vi "Create Key Index Map.vi"(6 "Key Map Transposed Primitive":refnum<class "2D Array u32.lvclass">, 8 "error in (no error)":errorcluster, 9 "Key Map Primitive":refnum<class "2D Array u32.lvclass">, 10 "Reduced Keys for Each line Profile":refnum<class "1D Array u32.lvclass">, 11 "Unique Keys":refnum<class "1D Array u32.lvclass">) -> (0 "error out":errorcluster, 3 "Key Line Profile Indexes":refnum<class "1D Array u32.lvclass">)   [LabVIEW 2024, in "G2CPU Line Profile.lvlib"]
uses:
  G2CPU Line Profile.lvlib
  <vilib>/Natan Biesmans/G2CPU GPU and CPU HPC Toolkit/G2CPU Libraries/Arrays/2DArray/u32/2D Array u32.lvclass
  C:/Program Files/National Instruments/LabVIEW 2025/vi.lib/Natan Biesmans/G2CPU GPU and CPU HPC Toolkit/G2CPU Libraries/Arrays/Array/Array Prototype.lvclass
  <vilib>/Natan Biesmans/G2CPU GPU and CPU HPC Toolkit/G2CPU Libraries/Arrays/1DArray/u32/1D Array u32.lvclass
  e7eb75a7-683b-4233-a57f-280f24811019.vi
  51fefef7-bdde-4c46-8d2b-12c633bde53a.vi
  0bb242c6-28a8-437e-9306-958441be214a.vi
  2070433c-6d53-4609-8e76-c76c78c5d5f5.vi
  18560914-5405-4c7e-9e60-f5c43eeeaa40.vi
  95130064-5133-4fc6-b00c-6381fdedbc79.vi
  e7eb75a7-683b-4233-a57f-280f24811019.vi/5793b77b-c002-4ebf-9075-685617c95341.vi
  e7eb75a7-683b-4233-a57f-280f24811019.vi/2ed3ef86-c00d-4d71-b84c-20267a6dfcf9.vi
  51fefef7-bdde-4c46-8d2b-12c633bde53a.vi/e9bebd79-1c27-4fc1-b91f-30516104c7f0.vi
  0bb242c6-28a8-437e-9306-958441be214a.vi/5793b77b-c002-4ebf-9075-685617c95341.vi
  0bb242c6-28a8-437e-9306-958441be214a.vi/2ed3ef86-c00d-4d71-b84c-20267a6dfcf9.vi
  2070433c-6d53-4609-8e76-c76c78c5d5f5.vi/e2b7cdad-9748-47a9-8803-19dad6ab3e2b.vi
  2070433c-6d53-4609-8e76-c76c78c5d5f5.vi/edeb7e37-ba5b-4522-b7cc-59d3333e22dd.vi
  18560914-5405-4c7e-9e60-f5c43eeeaa40.vi/7467a0f1-0650-4e63-b635-b3d2b2ec9a4e.vi
  18560914-5405-4c7e-9e60-f5c43eeeaa40.vi/8ee11bc3-5ef5-497e-97f0-8db2b3aaa149.vi
  18560914-5405-4c7e-9e60-f5c43eeeaa40.vi/c7af9698-5e3c-4e11-95da-3024075b67d2.vi
  95130064-5133-4fc6-b00c-6381fdedbc79.vi/a7ec311c-7cd8-4650-9526-d70ff0a769d1.vi
  e7eb75a7-683b-4233-a57f-280f24811019.vi/5793b77b-c002-4ebf-9075-685617c95341.vi/3e802c67-fb96-46a3-ae13-4994a8508b4f.vi
  e7eb75a7-683b-4233-a57f-280f24811019.vi/5793b77b-c002-4ebf-9075-685617c95341.vi/5a50fc67-79e7-4972-80c2-92243cd53dd4.vi
  e7eb75a7-683b-4233-a57f-280f24811019.vi/2ed3ef86-c00d-4d71-b84c-20267a6dfcf9.vi/730f6c57-5c0b-4ee9-b61e-75067b25222b.vi
  e7eb75a7-683b-4233-a57f-280f24811019.vi/2ed3ef86-c00d-4d71-b84c-20267a6dfcf9.vi/096b8799-7810-404e-baca-ba9279cec4bd.vi
  e7eb75a7-683b-4233-a57f-280f24811019.vi/2ed3ef86-c00d-4d71-b84c-20267a6dfcf9.vi/0f1a5a47-bcc5-4796-ac31-8dfcfbc0d7d1.vi
  e7eb75a7-683b-4233-a57f-280f24811019.vi/2ed3ef86-c00d-4d71-b84c-20267a6dfcf9.vi/89f12e17-3330-4b72-ad8f-8dd636660732.vi
  0bb242c6-28a8-437e-9306-958441be214a.vi/5793b77b-c002-4ebf-9075-685617c95341.vi/3e802c67-fb96-46a3-ae13-4994a8508b4f.vi
  0bb242c6-28a8-437e-9306-958441be214a.vi/5793b77b-c002-4ebf-9075-685617c95341.vi/5a50fc67-79e7-4972-80c2-92243cd53dd4.vi
  0bb242c6-28a8-437e-9306-958441be214a.vi/2ed3ef86-c00d-4d71-b84c-20267a6dfcf9.vi/730f6c57-5c0b-4ee9-b61e-75067b25222b.vi
  0bb242c6-28a8-437e-9306-958441be214a.vi/2ed3ef86-c00d-4d71-b84c-20267a6dfcf9.vi/096b8799-7810-404e-baca-ba9279cec4bd.vi
  0bb242c6-28a8-437e-9306-958441be214a.vi/2ed3ef86-c00d-4d71-b84c-20267a6dfcf9.vi/0f1a5a47-bcc5-4796-ac31-8dfcfbc0d7d1.vi
  0bb242c6-28a8-437e-9306-958441be214a.vi/2ed3ef86-c00d-4d71-b84c-20267a6dfcf9.vi/89f12e17-3330-4b72-ad8f-8dd636660732.vi
  2070433c-6d53-4609-8e76-c76c78c5d5f5.vi/e2b7cdad-9748-47a9-8803-19dad6ab3e2b.vi/edd31282-7992-4bba-af75-482693dee5e1.vi
  0bb242c6-28a8-437e-9306-958441be214a.vi/2ed3ef86-c00d-4d71-b84c-20267a6dfcf9.vi/730f6c57-5c0b-4ee9-b61e-75067b25222b.vi/0070e0fe-4ad7-4a3e-8965-d64becb7e5f0.vi
  <vilib>/Natan Biesmans/G2CPU GPU and CPU HPC Toolkit/G2CPU Libraries/Arrays/2DArray/binary/2D Array binary.lvclass
  <vilib>/Natan Biesmans/G2CPU GPU and CPU HPC Toolkit/G2CPU Libraries/Arrays/1DArray/binary/1D Array binary.lvclass
  <vilib>/Natan Biesmans/G2CPU GPU and CPU HPC Toolkit/G2CPU Libraries/Arrays/SubVI/Lock Arrays.vi
  <vilib>/Natan Biesmans/G2CPU GPU and CPU HPC Toolkit/G2CPU Libraries/Arrays/Array/G2CPU Get Array Pointer.vi
  <vilib>/Natan Biesmans/G2CPU GPU and CPU HPC Toolkit/G2CPU Libraries/Arrays/SubVI/is 2D.vi
  <vilib>/Natan Biesmans/G2CPU GPU and CPU HPC Toolkit/ArrayFire Driver/VIs/add.vi
  <vilib>/Natan Biesmans/G2CPU GPU and CPU HPC Toolkit/G2CPU Libraries/Arrays/Array/G2CPU Set Array Pointer.vi
  <vilib>/Natan Biesmans/G2CPU GPU and CPU HPC Toolkit/G2CPU Libraries/Arrays/Array/G2CPU Unlock Array.vi
  <vilib>/Natan Biesmans/G2CPU GPU and CPU HPC Toolkit/G2CPU Libraries/Arrays/Array/G2CPU Release Array.vi
  <vilib>/Natan Biesmans/G2CPU GPU and CPU HPC Toolkit/G2CPU Libraries/Arrays/Array/G2CPU Lock Array.vi
  <vilib>/Natan Biesmans/G2CPU GPU and CPU HPC Toolkit/ArrayFire Driver/VIs/transpose.vi
  <vilib>/Natan Biesmans/G2CPU GPU and CPU HPC Toolkit/ArrayFire Driver/VIs/eq.vi
  <vilib>/Natan Biesmans/G2CPU GPU and CPU HPC Toolkit/ArrayFire Driver/VIs/flat.vi
  <vilib>/Natan Biesmans/G2CPU GPU and CPU HPC Toolkit/ArrayFire Driver/VIs/where.vi
  <vilib>/Natan Biesmans/G2CPU GPU and CPU HPC Toolkit/G2CPU Libraries/Arrays/Array/Array Prototype.lvclass
  <vilib>/Natan Biesmans/G2CPU GPU and CPU HPC Toolkit/G2CPU Libraries/Arrays/DataTypes/U32/U32.lvclass
  <vilib>/Natan Biesmans/G2CPU GPU and CPU HPC Toolkit/G2CPU Libraries/Arrays/2DArray/2D Array Prototype.lvclass
  <vilib>/Natan Biesmans/G2CPU GPU and CPU HPC Toolkit/G2CPU Libraries/Arrays/1DArray/1D Array Prototype.lvclass
  <vilib>/Natan Biesmans/G2CPU GPU and CPU HPC Toolkit/G2CPU Libraries/Arrays/DataTypes/Boolean/Boolean.lvclass
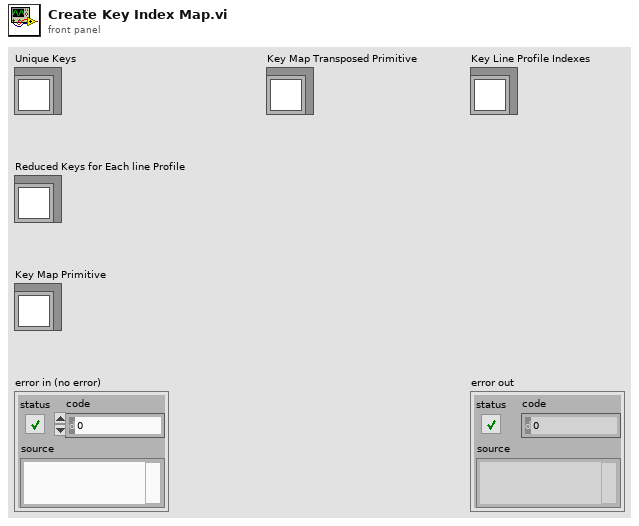
[diagram p1: front panel]
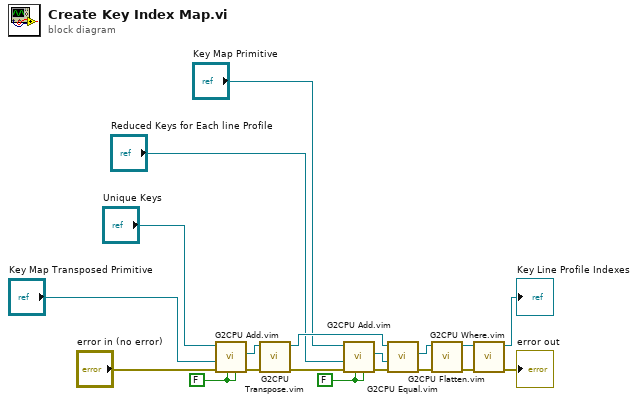
[diagram p0: block diagram]
diagram:
  w19 = FALSE ("Auto Release rhs (Enabled)")
  w12 = FALSE ("Auto Release lhs (Enabled)")
  n1 = call "G2CPU Add.vim"("Auto Release rhs (Enabled)"=w19, "Auto Release lhs (Enabled)"=w19, "error in (no error)"="error in (no error)", "Array rhs"="Key Map Transposed Primitive", "Array lhs"="Unique Keys") -> ("error out"=w7:errorcluster, "Array Result"=w9:refnum<class "2D Array u32.lvclass">)  [unwired: 5 in]
  n2 = call "G2CPU Transpose.vim"("error in (no error)"=w7, "Array In"=w9) -> ("error out"=w8:errorcluster, "Array out"=w11:refnum<class "2D Array u32.lvclass">)  [unwired: 8 in]
  n3 = call "G2CPU Add.vim"("Auto Release rhs (Enabled)"=w12, "Auto Release lhs (Enabled)"=w12, "error in (no error)"=w8, "Array rhs"="Reduced Keys for Each line Profile", "Array lhs"="Key Map Primitive") -> ("error out"=w17:errorcluster, "Array Result"=w5:refnum<class "2D Array u32.lvclass">)  [unwired: 5 in]
  n4 = call "G2CPU Equal.vim"("error in (no error)"=w17, "Array rhs"=w5, "Array lhs"=w11) -> ("error out"=w14:errorcluster, "Array Result"=w13:refnum<class "2D Array binary.lvclass">)  [unwired: 7 in]
  n5 = call "G2CPU Flatten.vim"("error in (no error)"=w14, "Array In"=w13) -> ("error out"=w16:errorcluster, "Array out"=w15:refnum<class "1D Array binary.lvclass">)  [unwired: 8 in]
  n6 = call "G2CPU Where.vim"("error in (no error)"=w16, "Array in"=w15) -> ("error out"=→"error out":errorcluster, "Non Zero Indices"=→"Key Line Profile Indexes":refnum<class "1D Array u32.lvclass">)  [unwired: 8 in]
